vi "test_libssh2_channel_get_exit_status.vi"() -> ()   [LabVIEW 2017, in "integration_tests.lvlib"]
uses:
  integration_tests.lvlib
  libssh2/libssh2_channel_open_ex.vi
  libssh2/libssh2_channel_process_startup.vi
  support/support.lvlib
  libssh2/libssh2.lvlib
  <vilib>/PNR/Transparent Assertions/Transparent Assertions/Transparent Assertions.lvlib
panel:
  out "error out":errorcluster
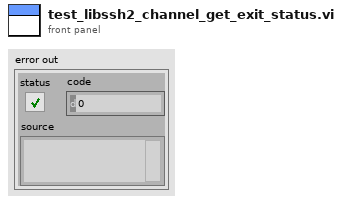
[diagram p1: front panel]
types:
  T1 = typedef "libssh2.lvlib/Session Refnum.ctl" = refnum<k1>
  T2 = typedef "libssh2.lvlib/Channel Refnum.ctl" = refnum<k1>
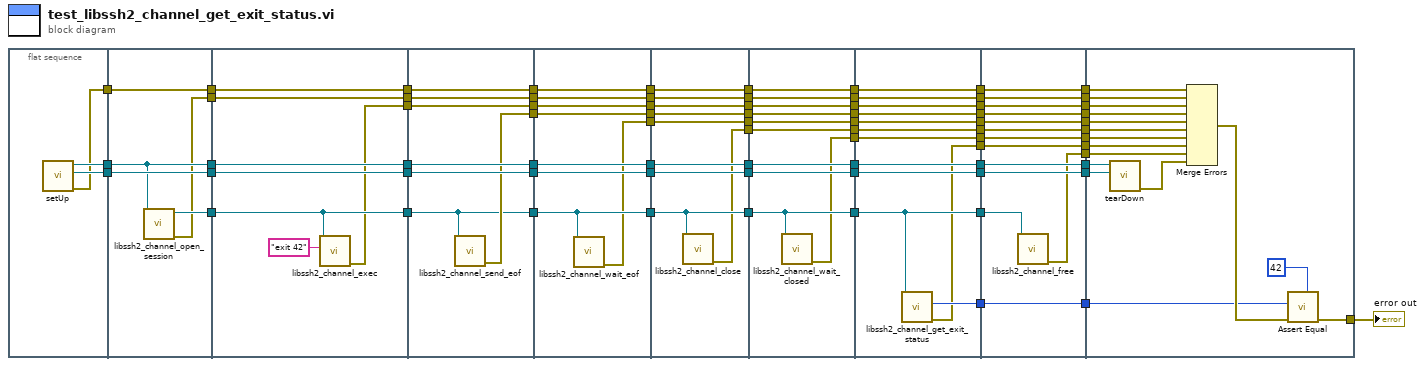
[diagram p0: block diagram]
diagram:
  n1 = flat-sequence {
    tunnel: [w76] -> w73
    tunnel: [w75] -> w72
    tunnel: [w74] -> w71
    tunnel: w73 -> [w80]
    tunnel: w72 -> [w81]
    tunnel: [w80] -> w70
    tunnel: [w81] -> w69
    tunnel: [w79] -> w68
    tunnel: w71 -> [w78]
    tunnel: [w78] -> w67
    tunnel: [w77] -> w66
    tunnel: w70 -> [w88]
    tunnel: [w88] -> w65
    tunnel: w69 -> [w87]
    tunnel: [w87] -> w64
    tunnel: w68 -> [w84]
    tunnel: [w84] -> w63
    tunnel: w67 -> [w86]
    tunnel: [w86] -> w62
    tunnel: w66 -> [w83]
    tunnel: [w83] -> w61
    tunnel: [w82] -> w60
    tunnel: w65 -> [w95]
    tunnel: [w95] -> w38
    tunnel: w64 -> [w94]
    tunnel: [w94] -> w36
    tunnel: w63 -> [w89]
    tunnel: [w89] -> w34
    tunnel: w62 -> [w93]
    tunnel: [w93] -> w32
    tunnel: w61 -> [w92]
    tunnel: [w92] -> w30
    tunnel: w60 -> [w91]
    tunnel: [w91] -> w28
    tunnel: [w90] -> w26
    tunnel: w38 -> [w103]
    tunnel: [w103] -> w37
    tunnel: w36 -> [w102]
    tunnel: [w102] -> w35
    tunnel: w34 -> [w97]
    tunnel: [w97] -> w33
    tunnel: w32 -> [w101]
    tunnel: [w101] -> w31
    tunnel: w30 -> [w100]
    tunnel: [w100] -> w29
    tunnel: w28 -> [w99]
    tunnel: [w99] -> w27
    tunnel: w26 -> [w98]
    tunnel: [w98] -> w25
    tunnel: [w96] -> w24
    tunnel: w37 -> [w112]
    tunnel: w35 -> [w111]
    tunnel: w33 -> [w110]
    tunnel: [w112] -> w21
    tunnel: [w111] -> w19
    tunnel: [w110] -> w17
    tunnel: [w109] -> w15
    tunnel: w31 -> [w108]
    tunnel: [w108] -> w13
    tunnel: w29 -> [w107]
    tunnel: [w107] -> w11
    tunnel: w27 -> [w106]
    tunnel: [w106] -> w9
    tunnel: w25 -> [w105]
    tunnel: [w105] -> w7
    tunnel: w24 -> [w104]
    tunnel: [w104] -> w5
    tunnel: w21 -> [w122]
    tunnel: [w122] -> w20
    tunnel: w19 -> [w121]
    tunnel: [w121] -> w18
    tunnel: w17 -> [w114]
    tunnel: [w114] -> w16
    tunnel: w15 -> [w120]
    tunnel: [w120] -> w14
    tunnel: w13 -> [w119]
    tunnel: [w119] -> w12
    tunnel: w11 -> [w118]
    tunnel: [w118] -> w10
    tunnel: w9 -> [w117]
    tunnel: [w117] -> w8
    tunnel: w7 -> [w116]
    tunnel: [w116] -> w6
    tunnel: w5 -> [w115]
    tunnel: [w115] -> w4
    tunnel: [w113] -> w3
    tunnel: w20 -> [w134]
    tunnel: [w134] -> w59
    tunnel: w18 -> [w133]
    tunnel: [w133] -> w58
    tunnel: w16 -> [w126]
    tunnel: [w126] -> w57
    tunnel: w14 -> [w132]
    tunnel: [w132] -> w56
    tunnel: w12 -> [w131]
    tunnel: [w131] -> w55
    tunnel: w10 -> [w130]
    tunnel: [w130] -> w54
    tunnel: w8 -> [w129]
    tunnel: [w129] -> w53
    tunnel: w6 -> [w128]
    tunnel: [w128] -> w52
    tunnel: [w127] -> w51
    tunnel: [w125] -> w50
    tunnel: w4 -> [w124]
    tunnel: [w124] -> w23
    tunnel: w3 -> [w123]
    tunnel: [w123] -> w2
    tunnel: w59 -> [w147]
    tunnel: w58 -> [w146]
    tunnel: w57 -> [w145]
    tunnel: [w147] -> w49
    tunnel: [w146] -> w48
    tunnel: [w144] -> w47
    tunnel: w56 -> [w143]
    tunnel: [w143] -> w46
    tunnel: w55 -> [w142]
    tunnel: [w142] -> w45
    tunnel: w54 -> [w141]
    tunnel: [w141] -> w44
    tunnel: w53 -> [w140]
    tunnel: [w140] -> w43
    tunnel: w52 -> [w139]
    tunnel: [w139] -> w42
    tunnel: [w138] -> w41
    tunnel: w51 -> [w138]
    tunnel: w50 -> [w137]
    tunnel: [w137] -> w40
    tunnel: w23 -> [w136]
    tunnel: [w136] -> w22
    tunnel: w2 -> [w135]
    tunnel: [w135] -> w1
    tunnel: w49 -> [w163]
    tunnel: w48 -> [w162]
    tunnel: [w161] -> w39
    tunnel: w47 -> [w159]
    tunnel: w46 -> [w158]
    tunnel: w45 -> [w157]
    tunnel: w44 -> [w155]
    tunnel: w43 -> [w154]
    tunnel: w42 -> [w153]
    tunnel: w41 -> [w152]
    tunnel: w40 -> [w151]
    tunnel: w22 -> [w149]
    tunnel: w1 -> [w148]
    frame #0 {
      n2 = call "setUp.vi"() -> ("error out"=w74:errorcluster, "connection ID"=w75:refnum<k5>, "session"=w76:T1)  [unwired: 9 in]
    }
    frame #1 {
      n3 = call "libssh2_channel_open_session.vi"("session"=w80) -> ("error out"=w77:errorcluster, "channel"=w79:T2)  [unwired: 9 in]
    }
    frame #2 {
      n4 = call "libssh2_channel_exec.vi"("command"="exit 42", "channel"=w84) -> ("error out"=w82:errorcluster)  [unwired: 9 in]
    }
    frame #3 {
      n5 = call "libssh2_channel_send_eof.vi"("channel"=w89) -> ("error out"=w90:errorcluster)  [unwired: 10 in]
    }
    frame #4 {
      n6 = call "libssh2_channel_wait_eof.vi"("channel"=w97) -> ("error out"=w96:errorcluster)  [unwired: 10 in]
    }
    frame #5 {
      n7 = call "libssh2_channel_close.vi"("channel"=w110) -> ("error out"=w109:errorcluster)  [unwired: 10 in]
    }
    frame #6 {
      n8 = call "libssh2_channel_wait_closed.vi"("channel"=w114) -> ("error out"=w113:errorcluster)  [unwired: 10 in]
    }
    frame #7 {
      n9 = call "libssh2_channel_get_exit_status.vi"("channel"=w126) -> ("error out"=w125:errorcluster, "exit status"=w127:i32)  [unwired: 9 in]
    }
    frame #8 {
      n10 = call "libssh2_channel_free.vi"("channel"=w145) -> ("error out"=w144:errorcluster)  [unwired: 10 in]
    }
    frame #9 {
      n11 = call "tearDown.vi"("connection ID"=w162, "session"=w163) -> ("error out"=w160:errorcluster)  [unwired: 9 in]
      n12 = Merge Errors(w157, w155, w154, w153, w149, w158, w148, w151, w159, w160) -> (w156:errorcluster)
      n13 = call <vilib>:"Assert Equal.vi"("Expected"=42 ("exitsignal"), "error in (no error)"=w156, "Actual"=w152) -> ("error out"=w161:errorcluster)  [unwired: 8 in]
    }
  }
  "error out" <- w39
